vi "Get stack name.vi"(0 "Module?":bool, 1 "Baseplate Type":string, 3 "Institution":string="CM", 5 "Protoname (baselayer)":string, 9 "Geometry":string="XX-", 11 "Resolution":string="HD", 12 "Numeric":dbl=54.0, 13 "Sensor thickness":dbl=100.0, 14 "Hexaboard ROC version":string="X") -> (8 "Stack name":string="320-PH-F1-CM-0054")   [LabVIEW 2021, in "Stack.lvclass"]
uses:
  Stack.lvclass
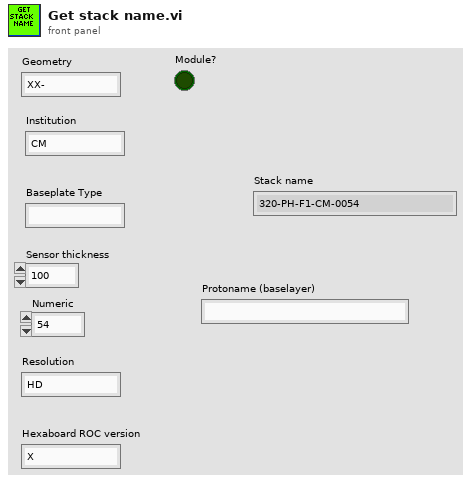
[diagram p1: front panel]
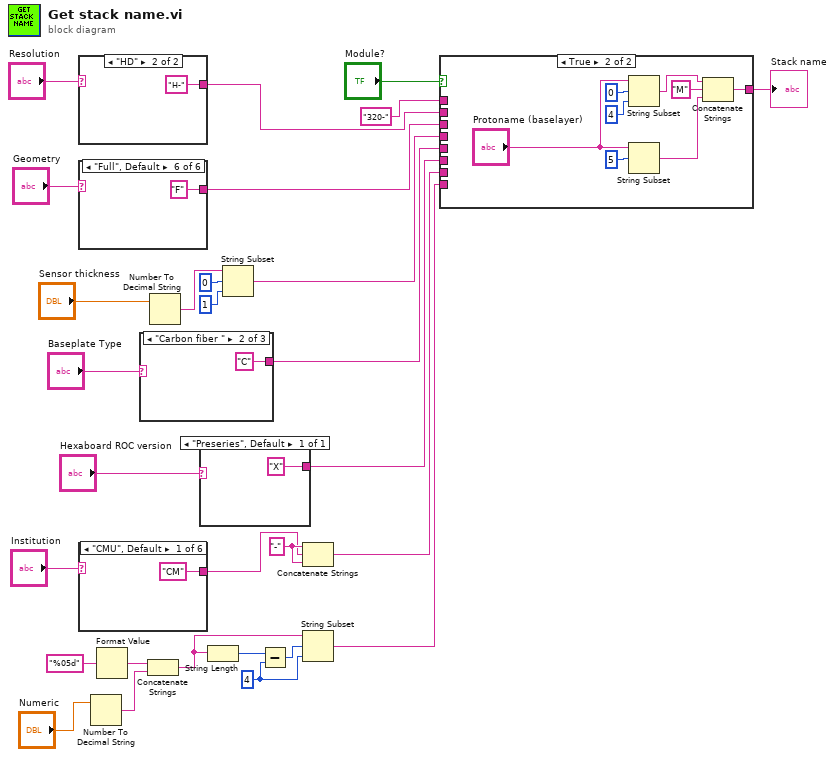
[diagram p0: block diagram]
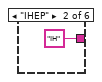
[diagram p2: hidden frame]
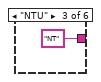
[diagram p3: hidden frame]
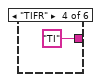
[diagram p4: hidden frame]
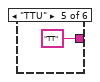
[diagram p5: hidden frame]
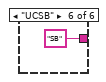
[diagram p6: hidden frame]
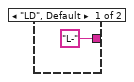
[diagram p7: hidden frame]
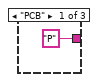
[diagram p8: hidden frame]
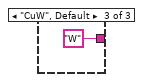
[diagram p9: hidden frame]
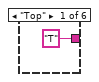
[diagram p10: hidden frame]
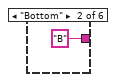
[diagram p11: hidden frame]
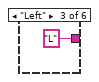
[diagram p12: hidden frame]
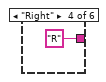
[diagram p13: hidden frame]
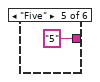
[diagram p14: hidden frame]
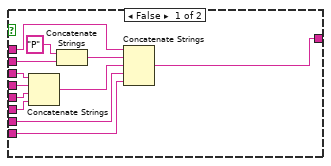
[diagram p15: hidden frame]
diagram:
  w17 = 4 ("length (rest)")
  w14 = "-" ("string")
  n1 = case shown="\"HD\"" "Resolution" {
    tunnel: ["L-" "H-"] -> w11
    frame "LD", Default {
    }
    frame "HD" {
    }
  }
  n2 = case shown="\"Full\", Default" "Geometry" {
    tunnel: ["T" "B" "L" "R" "5" "F"] -> w15
    frame "Top" {
    }
    frame "Bottom" {
    }
    frame "Left" {
    }
    frame "Right" {
    }
    frame "Five" {
    }
    frame "Full", Default {
    }
  }
  n3 = case shown="\"CMU\", Default" "Institution" {
    tunnel: ["CM" "IH" "NT" "TI" "TT" "SB"] -> w1
    frame "CMU", Default {
    }
    frame "IHEP" {
    }
    frame "NTU" {
    }
    frame "TIFR" {
    }
    frame "TTU" {
    }
    frame "UCSB" {
    }
  }
  n4 = Number To Decimal String(number="Numeric") -> (decimal integer string=w23:string)  [unwired: 1 in]
  n5 = Format Value(format string="%05d") -> (output string=w24:string)  [unwired: 2 in]
  n6 = case shown="\"Carbon fiber \"" "Baseplate Type" {
    tunnel: ["P" "C" "W"] -> w4
    frame "PCB" {
    }
    frame "Carbon fiber " {
    }
    frame "CuW", Default {
    }
  }
  n7 = Concatenate Strings(w24, w23) -> (w20:string)
  n8 = Number To Decimal String(number="Sensor thickness") -> (decimal integer string=w9:string)  [unwired: 1 in]
  n9 = case shown="\"Preseries\", Default" "Hexaboard ROC version" {
    tunnel: ["X"] -> w3
    frame "Preseries", Default {
    }
  }
  n10 = String Length(string=w20) -> (length=w18:i32)
  n11 = String Subset(string=w9, offset (0)=0, length (rest)=1 ("length (rest)")) -> (substring=w7:string)
  n12 = Subtract(x=w18, y=w17) -> (x-y=w19:i32)
  n13 = Concatenate Strings(w14, w1, w14) -> (w26:string)
  n14 = String Subset(string=w20, offset (0)=w19, length (rest)=w17) -> (substring=w21:string)
  n15 = case shown="True" "Module?" {
    tunnel: [w57 w67] -> w22
    tunnel: "320-" -> [w59 _]
    tunnel: w26 -> [w53 _]
    tunnel: w15 -> [w52 _]
    tunnel: w21 -> [w58 _]
    tunnel: w11 -> [w50 _]
    tunnel: w7 -> [w54 _]
    tunnel: w4 -> [w49 _]
    tunnel: w3 -> [w48 _]
    frame False {
      n16 = Concatenate Strings(w52, w54, w49, w48) -> (w51:string)
      n17 = Concatenate Strings("P", w50) -> (w55:string)
      n18 = Concatenate Strings(w59, w55, w51, w53, w58) -> (w57:string)
    }
    frame True {
      n19 = String Subset(string="Protoname (baselayer)", offset (0)=0, length (rest)=4 ("length (rest)")) -> (substring=w64:string)
      n20 = String Subset(string="Protoname (baselayer)", offset (0)=5) -> (substring=w61:string)  [unwired: 1 in]
      n21 = Concatenate Strings(w64, "M" ("string"), w61) -> (w67:string)
    }
  }
  "Stack name" <- w22
